vi "Write Data To Stop Bit.vi"(8 "error in (no error)":errorcluster, 10 "Stop Bit":bool, 11 "Generic Card in":refnum<class "Generic Card.lvclass">) -> (0 "error out":errorcluster, 3 "Generic Card out":refnum<class "Generic Card.lvclass">)   [LabVIEW 2014, in "Generic Instrument.lvlib" / "Generic Card.lvclass"]
uses:
  Generic Card.lvclass
  Generic Card.lvclass/Generic Card.ctl
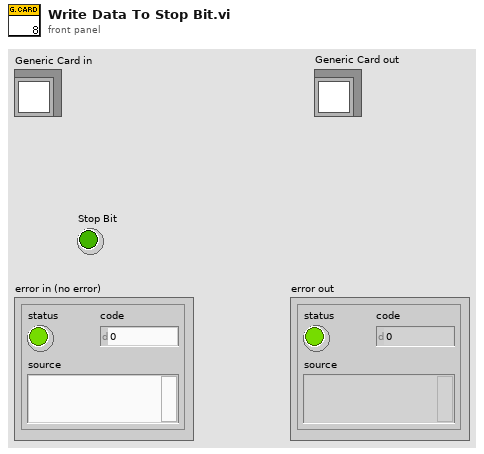
[diagram p1: front panel]
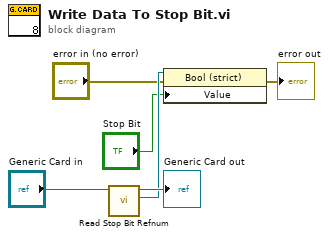
[diagram p0: block diagram]
diagram:
  n1 = call "Read Stop Bit Refnum.vi"("Generic Card in"="Generic Card in") -> ("Stop Bit Refnum"=w4:refnum<vi>, "Generic Card out"=→"Generic Card out":refnum<class "Generic Card.lvclass">)  [unwired: 8 in, 1 out]
  n2 = property class="Bool (strict)"(reference=w4, error in="error in (no error)", "Value"="Stop Bit") -> (error out=→"error out":errorcluster)  [unwired: 1 out]
